vi "Try Parse.vi"(0 "SG Path in":refnum<class "SG Path.lvclass">, 5 "Config Row":string[](array[string]), 11 "error in":errorcluster) -> (4 "SG Path out":refnum<class "SG Path.lvclass">, 6 "Is of type?":bool, 15 "error out":errorcluster)   [LabVIEW 2023, in "RFFixtureCharact.Public.lvlib" / "SG Path.lvclass"]
uses:
  SG Path.lvclass
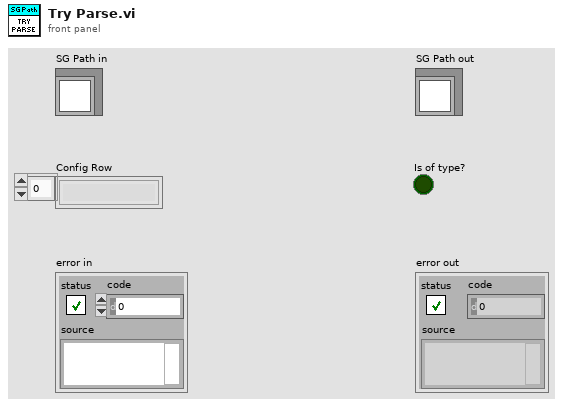
[diagram p1: front panel]
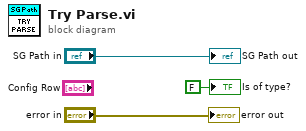
[diagram p0: block diagram]
diagram:
  "error out" <- "error in"
  "SG Path out" <- "SG Path in"
  "Is of type?" <- FALSE ("Is of type?")
